vi "Set Cell Value (SharedString).vi"(6 "Value":string, 8 "error in":errorcluster, 9 "Cell Address":string, 10 "WorksheetPart":refnum<k24>, 11 "SpreadsheetDoc in":refnum<k24>) -> (0 "error out":errorcluster, 2 "WorksheetPart out":refnum<k24>, 3 "SpreadsheetDoc out":refnum<k24>)   [LabVIEW 2019, in "Open Xml.lvlib"]
uses:
  Open Xml.lvlib
  D:/git/Open-Xml-LabVIEW/Source/DocumentFormat.OpenXml.dll
  DocumentFormat.OpenXml.dll
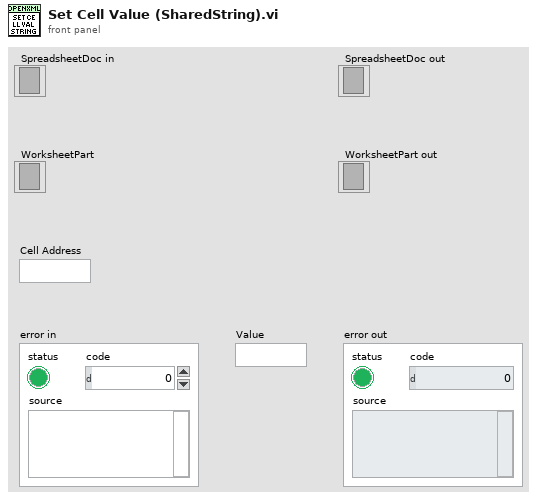
[diagram p1: front panel]
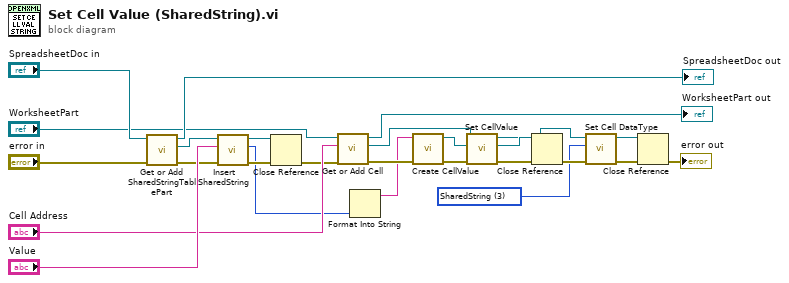
[diagram p0: block diagram]
diagram:
  w19 = 3 items=["Boolean", "Number", "Error", "SharedString", "String", "InlineString", "Date"] ("Datatype")
  n1 = call "Get or Add SharedStringTablePart.vi"("error in"="error in", "SpreadsheetDoc in"="SpreadsheetDoc in") -> ("error out"=w3:errorcluster, "SharedStringTablePart"=w2:refnum<k24>, "SpreadsheetDoc out"=→"SpreadsheetDoc out":refnum<k24>)  [unwired: 7 in]
  n2 = call "Insert SharedString.vi"("error in"=w3, "Value"="Value", "SharedStringTablePart in"=w2) -> ("error out"=w13:errorcluster, "Index"=w10:i32, "SharedStringTablePart out"=w12:refnum<k24>)  [unwired: 6 in]
  n3 = Close Reference(reference=w12, error in (no error)=w13) -> (error out=w11:errorcluster)
  n4 = call "Get or Add Cell.vi"("error in"=w11, "Cell Address"="Cell Address", "Worksheetpart in"="WorksheetPart") -> ("error out"=w6:errorcluster, "Cell"=w14:refnum<k24>, "WorksheetPart out"=→"WorksheetPart out":refnum<k24>)  [unwired: 6 in]
  n5 = Format Into String(w10) -> (resulting string=w5:string)  [unwired: 3 in, 1 out]
  n6 = call "Create CellValue.vi"("error in"=w6, "Text"=w5) -> ("error out"=w7:errorcluster, "CellValue out"=w22:refnum<k24>)  [unwired: 8 in]
  n7 = call "Set CellValue.vi"("error in"=w7, "CellValue in"=w22, "Cell in"=w14) -> ("error out"=w20:errorcluster, "CellValue out"=w26:refnum<k24>, "Cell out"=w8:refnum<k24>)  [unwired: 6 in]
  n8 = Close Reference(reference=w26, error in (no error)=w20) -> (error out=w25:errorcluster)
  n9 = call "Set Cell DataType.vi"("error in"=w25, "Datatype"=w19, "Cell in"=w8) -> ("error out"=w9:errorcluster, "Cell out"=w24:refnum<k24>)  [unwired: 7 in]
  n10 = Close Reference(reference=w24, error in (no error)=w9) -> (error out=→"error out":errorcluster)
